vi "tra25cc_get_status.vi"(8 "error in (no error)":errorcluster, 11 "conn_xyz_in":T4) -> (0 "error out":errorcluster, 1 "position_xyz":cluster{"pos_x":dbl, "pos_y":dbl, "pos_z":dbl}, 2 "state_xyz":T2, 3 "conn_xyz_out":T3, 4 "current_speed_xyz":T1)   [LabVIEW 2014]
uses:
  \\CL3-USR4\usr4/F103625/Scanner_v3_current/src/Stage_xyz/Dll/Newport.CONEXCC.CommandInterface.dll
  Dll/Newport.CONEXCC.CommandInterface.dll
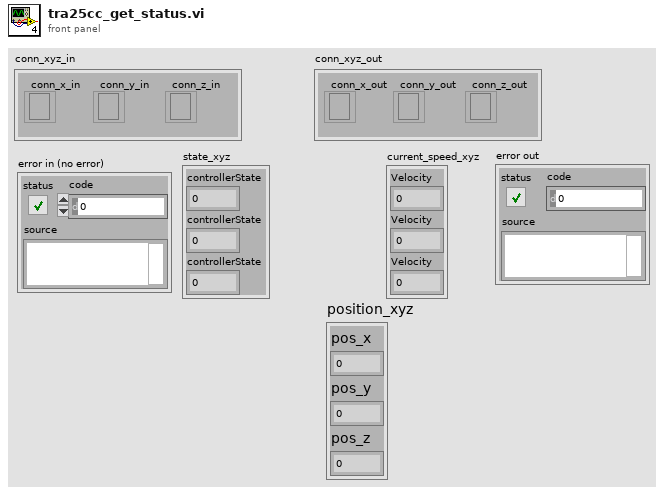
[diagram p1: front panel]
types:
  T1 = cluster{"Velocity":dbl, "Velocity":dbl, "Velocity":dbl}
  T2 = cluster{"controllerState":u32, "controllerState":u32, "controllerState":u32}
  T3 = cluster{"conn_x_out":refnum<k24>, "conn_y_out":refnum<k24>, "conn_z_out":refnum<k24>}
  T4 = cluster{"conn_x_in":refnum<k24>, "conn_y_in":refnum<k24>, "conn_z_in":refnum<k24>}
  T5 = cluster{"controllerState":string, "controllerState":string, "controllerState":string}
  T6 = cluster{"CurrentPosition":dbl, "CurrentPosition":dbl, "CurrentPosition":dbl}
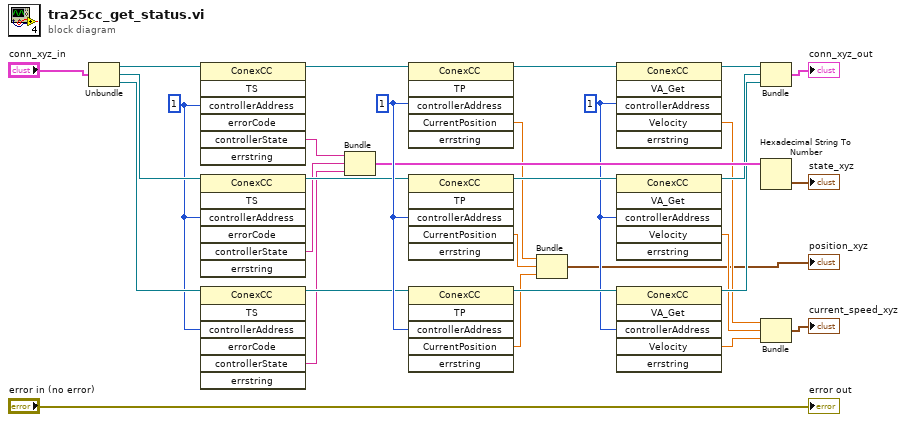
[diagram p0: block diagram]
diagram:
  w10 = 1 ("controllerAddress")
  w26 = 1 ("controllerAddress")
  w25 = 1 ("controllerAddress")
  n1 = Unbundle("conn_xyz_in") -> ("conn_x_in"=w30:refnum<k24>, "conn_y_in"=w29:refnum<k24>, "conn_z_in"=w28:refnum<k24>)
  n2 = invoke class="ConexCC" method="TS"(reference=w30, "controllerAddress"=w25) -> (reference out=w24:refnum<k24>, "controllerState"=w20:string)  [unwired: 5 in, 5 out]
  n3 = invoke class="ConexCC" method="TS"(reference=w29, "controllerAddress"=w25) -> (reference out=w23:refnum<k24>, "controllerState"=w19:string)  [unwired: 5 in, 5 out]
  n4 = invoke class="ConexCC" method="TS"(reference=w28, "controllerAddress"=w25) -> (reference out=w22:refnum<k24>, "controllerState"=w18:string)  [unwired: 5 in, 5 out]
  n5 = Bundle("controllerState"=w20, "controllerState"=w19, "controllerState"=w18) -> (w17:T5)  [unwired: 1 in]
  n6 = invoke class="ConexCC" method="TP"(reference=w24, "controllerAddress"=w26) -> (reference out=w16:refnum<k24>, "CurrentPosition"=w4:dbl)  [unwired: 4 in, 4 out]
  n7 = invoke class="ConexCC" method="TP"(reference=w23, "controllerAddress"=w26) -> (reference out=w14:refnum<k24>, "CurrentPosition"=w3:dbl)  [unwired: 4 in, 4 out]
  n8 = invoke class="ConexCC" method="TP"(reference=w22, "controllerAddress"=w26) -> (reference out=w12:refnum<k24>, "CurrentPosition"=w2:dbl)  [unwired: 4 in, 4 out]
  n9 = Bundle("CurrentPosition"=w4, "CurrentPosition"=w3, "CurrentPosition"=w2) -> (→"position_xyz":T6)  [unwired: 1 in]
  n10 = invoke class="ConexCC" method="VA_Get"(reference=w16, "controllerAddress"=w10) -> (reference out=w15:refnum<k24>, "Velocity"=w7:dbl)  [unwired: 4 in, 4 out]
  n11 = invoke class="ConexCC" method="VA_Get"(reference=w14, "controllerAddress"=w10) -> (reference out=w13:refnum<k24>, "Velocity"=w8:dbl)  [unwired: 4 in, 4 out]
  n12 = invoke class="ConexCC" method="VA_Get"(reference=w12, "controllerAddress"=w10) -> (reference out=w11:refnum<k24>, "Velocity"=w9:dbl)  [unwired: 4 in, 4 out]
  n13 = Bundle("conn_x_in"=w15, "conn_y_in"=w13, "conn_z_in"=w11) -> (→"conn_xyz_out":T4)  [unwired: 1 in]
  n14 = Hexadecimal String To Number(string=w17) -> (number=→"state_xyz":T2)  [unwired: 2 in, 1 out]
  n15 = Bundle("Velocity"=w7, "Velocity"=w8, "Velocity"=w9) -> (→"current_speed_xyz":T1)  [unwired: 1 in]
  "error out" <- "error in (no error)"
